vi "Set Plot Names.vi"(8 "entrée d'erreur (pas d'erreur)":errorcluster, 10 "Noms des tracés":string[](array[string]), 11 "Référence au graphe":refnum<vi>) -> (0 "sortie d'erreur":errorcluster)   [LabVIEW 2009]
doc: "Ce VI sert à définir le nom des tracés sur un graphe déroulant ou un graphe."
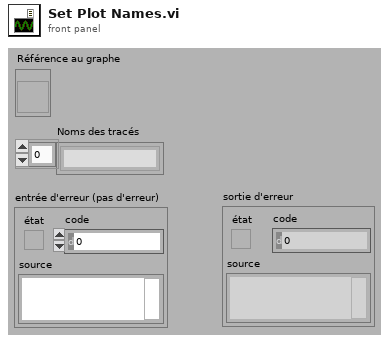
[diagram p1: front panel]
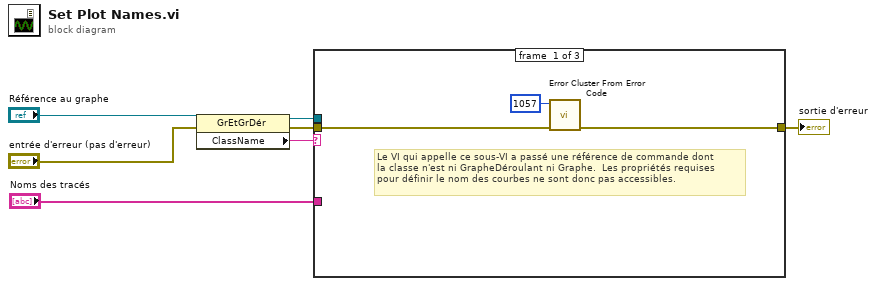
[diagram p0: block diagram]
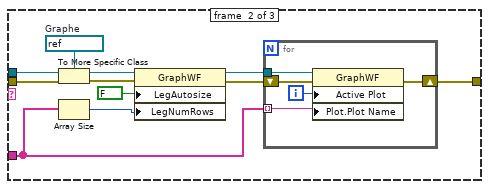
[diagram p2: hidden frame]
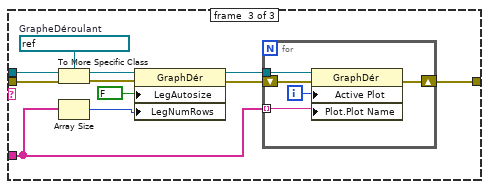
[diagram p3: hidden frame]
diagram:
  n1 = property on="Nœud de propriété" class="GrEtGrDér"(reference="Référence au graphe", error in="entrée d'erreur (pas d'erreur)") -> (reference out=w4:refnum<vi>, error out=w5:errorcluster, "ClassName"=w6:string)
  n2 = case "Structure Condition" shown="\"WaveformGraph\"" w6 {
    tunnel: w5 -> [w9 w15 w31]
    tunnel: w4 -> [_ w16 w32]
    tunnel: "Noms des tracés" -> [_ w11 w27]
    tunnel: [w8 w13 w29] -> w1
    frame #0 {
      # "Le VI qui appelle ce sous-VI a passé une référence de commande dont\nla classe n'est ni GrapheDéroulant ni Graphe.  Les propriétés requises\npour définir le nom des courbes ne sont donc pas accessibles."
      n3 = call <vilib>:"Error Cluster From Error Code.vi"("error in (no error)"=w9, "error code (0)"=1057) -> ("error out"=w8:errorcluster)  [unwired: 1 in, 6 out]
    }
    frame #1 {
      w21 = refnum<vi> refnum  # Graphe
      n4 = To More Specific Class(target class=w21, reference=w16, error in=w15) -> (specific class reference=w19:refnum<vi>, error out=w20:errorcluster)
      n5 = Array Size ("Taille d'un tableau")(array=w11) -> (size(s)=w12:i32)
      n6 = property on="Nœud de propriété" class="GraphWF"(reference=w19, error in=w20, "LegAutosize"=FALSE ("Legend:Autosize"), "LegNumRows"=w12) -> (reference out=w17:refnum<vi>, error out=w14:errorcluster)
      n7 = for "Boucle For" {
        tunnel: w17 -> [w26]
        shift-right: [w24] -> w13
        shift-left: w14 -> [w25]
        tunnel: w11 -> [w22] mode=indexing
        i -> [w23]
        n8 = property class="GraphWF"(reference=w26, error in=w25, "Active Plot"=w23, "Plot.Plot Name"=w22) -> (error out=w24:errorcluster)  [unwired: 1 out]
      }
    }
    frame #2 {
      w37 = refnum<vi> refnum  # GrapheDéroulant
      n9 = To More Specific Class(target class=w37, reference=w32, error in=w31) -> (specific class reference=w35:refnum<vi>, error out=w36:errorcluster)
      n10 = Array Size ("Taille d'un tableau")(array=w27) -> (size(s)=w28:i32)
      n11 = property on="Nœud de propriété" class="GraphDér"(reference=w35, error in=w36, "LegAutosize"=FALSE ("Legend:Autosize"), "LegNumRows"=w28) -> (reference out=w33:refnum<vi>, error out=w30:errorcluster)
      n12 = for "Boucle For" {
        tunnel: w33 -> [w42]
        shift-right: [w40] -> w29
        shift-left: w30 -> [w41]
        tunnel: w27 -> [w38] mode=indexing
        i -> [w39]
        n13 = property class="GraphDér"(reference=w42, error in=w41, "Active Plot"=w39, "Plot.Plot Name"=w38) -> (error out=w40:errorcluster)  [unwired: 1 out]
      }
    }
  }
  "sortie d'erreur" <- w1
